vi "SystemSet.vi"(7 "参数查询(0)/设置(1)":bool, 8 "error in (no error)":errorcluster caption="错误输入（无错误）", 9 "设置参数":string, 10 "SYSTEM命令子系统":string(combo), 11 "VISA资源名称":refnum<visa-resource-name>) -> (0 "error out":errorcluster caption="错误输出", 1 "查询返回字节数":u32, 2 "查询返回":string, 3 "VISA资源名称 2":refnum<visa-resource-name>)   [LabVIEW 2018]
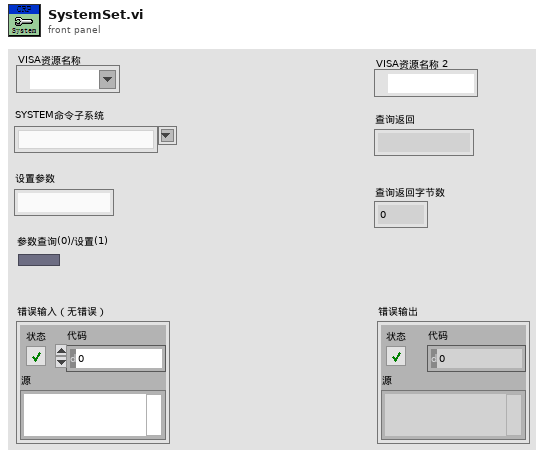
[diagram p1: front panel]
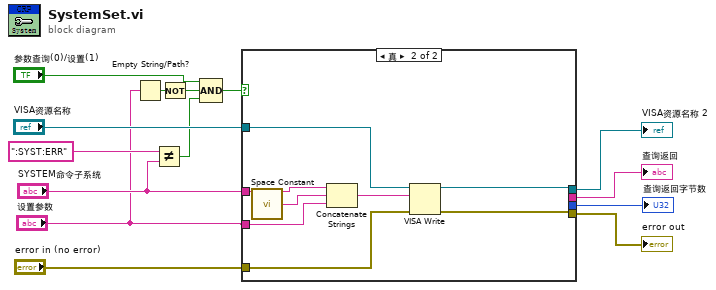
[diagram p0: block diagram]
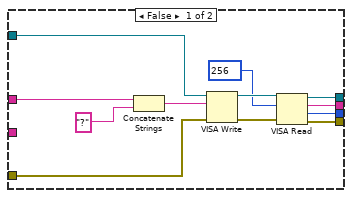
[diagram p2: hidden frame]
diagram:
  n1 = Empty String/Path?(string/path="设置参数") -> (empty?=w9:bool)
  n2 = Not Equal?(x=":SYST:ERR", y="SYSTEM命令子系统") -> (x != y?=w3:bool)
  n3 = Not(x=w9) -> (.not. x?=w1:bool)
  n4 = Compound Arithmetic op=AND ("复合运算")("参数查询(0)/设置(1)", w1, w3) -> (w8:bool)
  n5 = case shown="真" w8 {
    tunnel: "设置参数" -> [_ w34]
    tunnel: "SYSTEM命令子系统" -> [w26 w32]
    tunnel: "VISA资源名称" -> [w15 w31]
    tunnel: "error in (no error)" -> [w23 w29]
    tunnel: [w19 w28] -> w10
    tunnel: [w18 w27] -> w11
    tunnel: [w17 _] -> w12
    tunnel: [w16 _] -> w6
    frame False {
      n6 = Concatenate Strings(w26, "?" ("字符串")) -> (w24:string)
      n7 = VISA Write(VISA resource name=w15, write buffer=w24, error in (no error)=w23) -> (VISA resource name out=w22:refnum<visa-resource-name>, error out=w21:errorcluster)  [unwired: 1 out]
      n8 = VISA Read(VISA resource name=w22, byte count=u32 256 ("字节总数"), error in (no error)=w21) -> (VISA resource name out=w18:refnum<visa-resource-name>, read buffer=w17:string, return count=w16:u32, error out=w19:errorcluster)
    }
    frame True {
      n9 = call <vilib>:"Space Constant.vi"() -> ("String"=w33:string)
      n10 = Concatenate Strings(w32, w33, w34) -> (w30:string)
      n11 = VISA Write(VISA resource name=w31, write buffer=w30, error in (no error)=w29) -> (VISA resource name out=w27:refnum<visa-resource-name>, error out=w28:errorcluster)  [unwired: 1 out]
    }
  }
  "VISA资源名称 2" <- w11
  "error out" <- w10
  "查询返回" <- w12
  "查询返回字节数" <- w6
